vi "UTILITY Array Get 1D String Column From 2D.vi"(0 "2D Array Data":string[][](array[string]), 7 "column index":i32) -> (4 "Column Data":string[](array[string]))   [LabVIEW 2018]
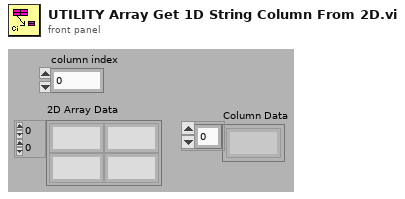
[diagram p1: front panel]
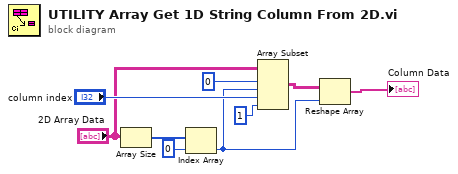
[diagram p0: block diagram]
diagram:
  n1 = Array Size(array="2D Array Data") -> (size(s)=w3:i32[])
  n2 = Index Array(array=w3, index=0) -> (element=w1:i32)
  n3 = Array Subset(array="2D Array Data", index (row)=0 ("index"), length (row)=w1, index (col)="column index", length (col)=1 ("length")) -> (w6:string[][])
  n4 = Reshape Array(w6, w1) -> (→"Column Data":string[])
